vi "BK Precision 1823A Data Logging.vi"() -> ()   [LabVIEW 2017]
doc: "This example demonstrates a fast way to log data into a text file using B&K Precision 1823A frequency counter."
uses:
  BK Precision 1823A.lvlib
panel:
  in  "Path":path
  in  "Select Function":i8(ring) items=["Frequency A", "Frequency B", "Frequency C", "Period", "Total", "Ratio", "T.I"]
  in  "Select Gate Time":i8(ring) items=["0.01", "0.1", "1", "10"]
  in  "stop":bool
  in  "Time Interval (1000)":u16=1000 min=100 step=1
  out "Measured Data Value":string
  in  "VISA resource name":refnum<visa-resource-name>
  # "(c) 2009 B&K PRECISION CORPORATION.  ALL RIGHTS RESERVED."
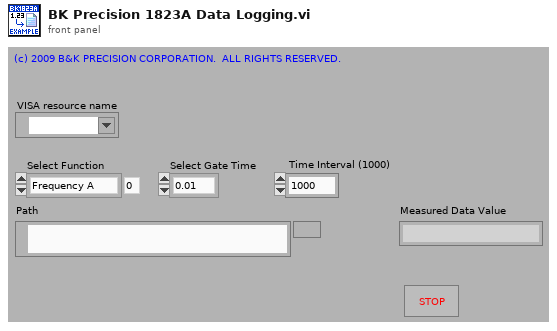
[diagram p1: front panel]
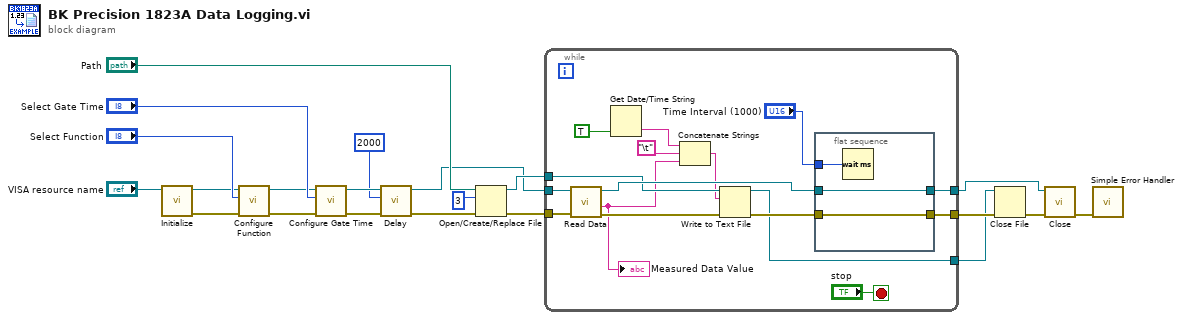
[diagram p0: block diagram]
diagram:
  n1 = call "Initialize.vi"("VISA resource name"="VISA resource name") -> ("error out"=w16:errorcluster, "VISA resource name out"=w17:refnum<visa-resource-name>)  [unwired: 9 in]
  n2 = call "Configure Function.vi"("error in (no error)"=w16, "Select Function (0)"="Select Function", "VISA resource name"=w17) -> ("error out"=w14:errorcluster, "VISA resource name out"=w15:refnum<visa-resource-name>)  [unwired: 7 in]
  n3 = call "Configure Gate Time.vi"("error in (no error)"=w14, "Select Gate Time (0.01)"="Select Gate Time", "VISA resource name"=w15) -> ("error out"=w5:errorcluster, "VISA resource name out"=w4:refnum<visa-resource-name>)  [unwired: 7 in]
  n4 = call "Delay.vi"("error in (no error)"=w5, "Delay Value (150)"=2000, "VISA resource name"=w4) -> ("error out"=w2:errorcluster, "VISA resource name out"=w3:refnum<visa-resource-name>)  [unwired: 7 in]
  n5 = Open/Create/Replace File(file path (use dialog)="Path", error in=w2, operation (0:open)=3) -> (refnum out=w13:refnum<file>, error out=w10:errorcluster)  [unwired: 3 in, 1 out]
  n6 = while {
    tunnel: [w35] -> w6
    tunnel: [w34] -> w9
    tunnel: w3 -> [w33]
    tunnel: w10 -> [w32]
    tunnel: w13 -> [w30]
    tunnel: [w26] -> w7
    stop <- "stop" stop-if-true
    n7 = call "Read Data.vi"("error in (no error)"=w32, "VISA resource name"=w33) -> ("error out"=w29:errorcluster, "Return String"=w24:string, "VISA resource name out"=w31:refnum<visa-resource-name>)  [unwired: 6 in, 1 out]
    "Measured Data Value" <- w24
    n8 = Get Date/Time String(want seconds? (F)=TRUE) -> (time string=w25:string)  [unwired: 2 in, 1 out]
    n9 = Concatenate Strings(w25, "\t", w24) -> (w27:string)
    n10 = Write to Text File(file (use dialog)=w30, text=w27, error in=w29) -> (refnum out=w26:refnum<file>, error out=w28:errorcluster)  [unwired: 1 in, 1 out]
    n11 = flat-sequence {
      tunnel: "Time Interval (1000)" -> [w40]
      tunnel: [w38] -> w35
      tunnel: [w39] -> w34
      tunnel: w28 -> [w39]
      tunnel: w31 -> [w38]
      frame #0 {
        n12 = Wait (ms)(milliseconds to wait=w40) -> ()  [unwired: 1 out]
      }
    }
  }
  n13 = Close File(refnum=w7, error in=w9) -> (error out=w8:errorcluster)  [unwired: 1 out]
  n14 = call "Close.vi"("error in (no error)"=w8, "VISA resource name"=w6) -> ("error out"=w21:errorcluster)  [unwired: 9 in]
  n15 = call <vilib>:"Simple Error Handler.vi"("error in (no error)"=w21) -> ()  [unwired: 4 in, 5 out]
